vi "optionsFrame_CppGlobals.vi"() -> ()   [LabVIEW 2016]
panel:
  out "#if NI_SECURITY_VI_SERVER":bool
  out "#if_RecentlyOpenedFiles":bool
  out "#if_MacX86":bool
  out "#if_Unix":bool
  out "#if_OLEServer":bool
  out "#if_WinCE":bool
  out "#if_UseNativeFileDialog":bool
  out "#if_XWindows":bool
  out "#if_MSWin":bool
  out "#if_UndoReady":bool
  out "#if_Sparc":bool
  out "#if_Mac":bool
  out "#if_AppLibs":bool
  out "#if_ThreadsUsed":bool
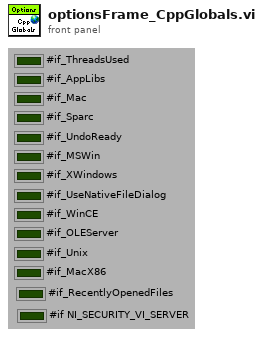
[diagram p1: front panel]
diagram:
